vi "To Cluster.vi"(7 "Tree ID":string, 8 "Error In":errorcluster, 10 "Cluster Type":variant, 11 "Tree Data Type":refnum<class "Tree Data.lvclass">) -> (0 "Error Out":errorcluster, 1 "Cluster Variant":variant, 3 "Tree Data Out":refnum<class "Tree Data.lvclass">)   [LabVIEW 2017, in "Tree API.lvlib" / "Tree.lvclass"]
doc: "Look at the Tree specified by Tree ID and try to extract data from it, following the structure of the wired cluster type. The names of cluster and their types must match those contained in the Tree. The Tree can contain more elements than the cluster. Only the default supported data types can be converted using this method. If your cluster contains anything more complicated than default Tree Data Types, you need to write your own low level cluster translation."
uses:
  Tree.lvclass
  Tree Data/Tree Data.lvclass
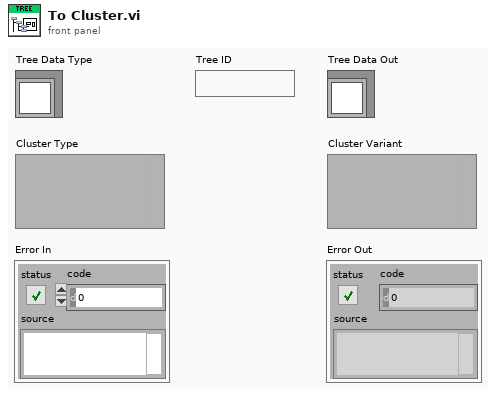
[diagram p1: front panel]
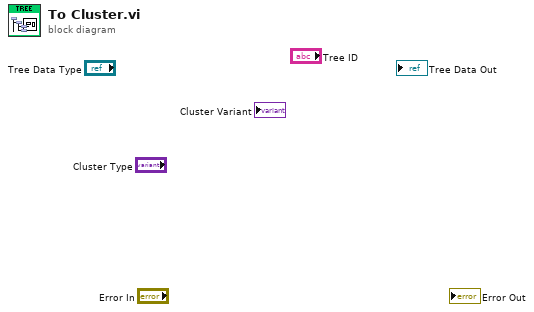
[diagram p0: block diagram]
diagram:
